vi "SetActorScalingDetailsRoomT.vi"(8 "error in":T2, 11 "Actor Scaling Details Room Temperature Input Cluster":T1={"xy Max Voltage"=-inf, "xy Max Range"=-inf, "z Max Voltage"=-inf, "z Max Range"=-inf} {"z Max Range" format="%#_g µm"; "z Max Voltage" format="%#_g V"; "xy Max Range" format="%#_g µm"; "xy Max Voltage" format="%#_g V"}) -> (0 "error out":T2, 3 "output cluster":T1={"xy Max Voltage"=-inf, "xy Max Range"=-inf, "z Max Voltage"=-inf, "z Max Range"=-inf} {"z Max Range" format="%#_g µm"; "z Max Voltage" format="%#_g V"; "xy Max Range" format="%#_g µm"; "xy Max Voltage" format="%#_g V"})   [LabVIEW 2016]
doc: "Specifies the details of the room temperature profile. The clusters contains the following variables:\n- x,y Max Voltage [V] (float)[1 to 10]\n- z Max Voltage [V] (float) [1 to 10]\n- x,y Max Range [µm] (float) [0 to 2000000]\n- z Max Range [µm] (float) [0 to 2000000]\nBy passing -Inf (float) or -2147483648 (integer) as input values, the corresponding parameter(s) will be read out."
uses:
  Controls/Error_Out.ctl
  Controls/ActorScalingDetailsRoomT_Parameters.ctl
  Files_ASC500/DLL/ASC500_RemoteControlV27.dll
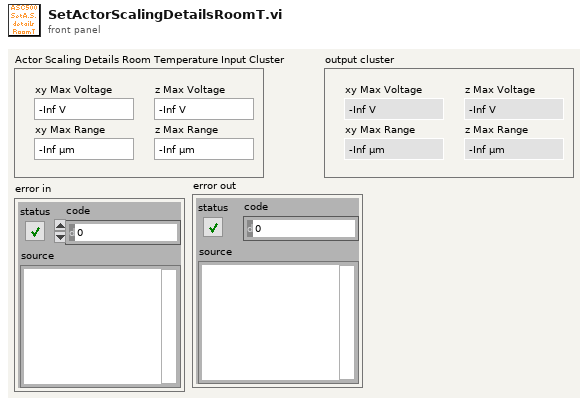
[diagram p1: front panel]
types:
  T1 = typedef "ActorScalingDetailsRoomT_Parameters.ctl" = cluster{"xy Max Voltage":dbl, "xy Max Range":dbl, "z Max Voltage":dbl, "z Max Range":dbl}
  T2 = typedef "Error_Out.ctl" = errorcluster
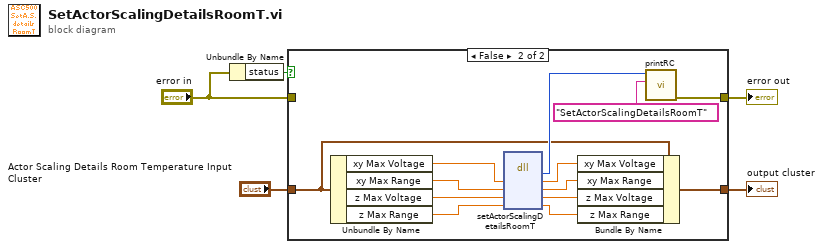
[diagram p0: block diagram]
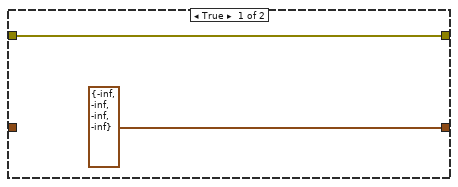
[diagram p2: hidden frame]
diagram:
  n1 = Unbundle By Name("error in") -> ("status"=w5:bool)
  n2 = case shown="False" w5 {
    tunnel: [w6 w20] -> w4
    tunnel: "Actor Scaling Details Room Temperature Input Cluster" -> [_ w13]
    tunnel: [T1 {"xy Max Voltage"=-inf, "xy Max Range"=-inf, "z Max Voltage"=-inf, "z Max Range"=-inf} ("Actor Scaling Details Room Temperature Input Cluster") w8] -> w2
    tunnel: "error in" -> [w6 _]
    frame True {
    }
    frame False {
      n3 = Unbundle By Name(w13) -> ("xy Max Voltage"=w17:dbl, "xy Max Range"=w16:dbl, "z Max Voltage"=w15:dbl, "z Max Range"=w14:dbl)
      n4 = dll-call lib="G:/SCMOperations/Share/ELE/Produkt Information/ASC500/04 Remote Control/02 development versions/2018Nov06/Files_ASC500/DLL/ASC500_RemoteControlV27.dll" fn="setActorScalingDetailsRoomT"("xy Max Voltage"=w17, "xy Max Range"=w16, "z Max Voltage"=w15, "z Max Range"=w14) -> ("RC"=w19:i32, "xy Max Voltage"=w12:sgl, "xy Max Range"=w11:sgl, "z Max Voltage"=w10:sgl, "z Max Range"=w9:sgl)  [unwired: 3 in, 2 out]
      n5 = Bundle By Name(cluster=w13, "xy Max Voltage"=w12, "xy Max Range"=w11, "z Max Voltage"=w10, "z Max Range"=w9) -> (w8:T1)
      n6 = call "printRC.vi"("additional information"="SetActorScalingDetailsRoomT", "RC"=w19) -> ("error out"=w20:T2)  [unwired: 9 in]
    }
  }
  "error out" <- w4
  "output cluster" <- w2
